vi "Exponential Smooth.vi"(10 "Smoothing Factor":dbl=0.1, 11 "Input Value":dbl) -> (3 "Smoothed Value":dbl)   [LabVIEW 2011]
doc: "Exponential smoothing weights the input value against the previous smoothing value.\n\nTODO: possible improvement: when there has been a long string of NaN inputs, we should probably disregard the old smoothed value and begin afresh."
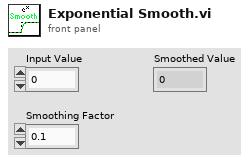
[diagram p1: front panel]
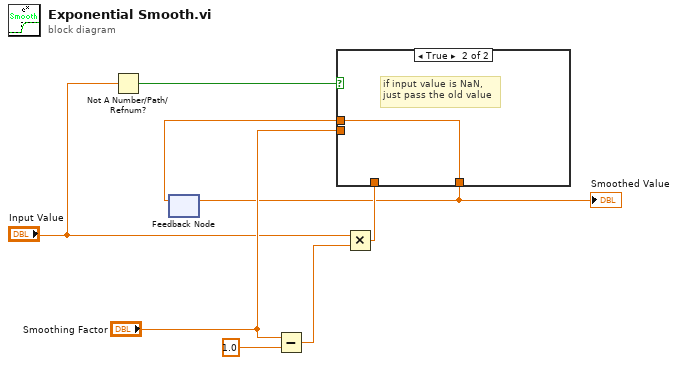
[diagram p0: block diagram]
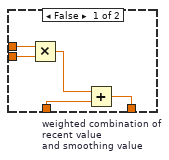
[diagram p2: hidden frame]
diagram:
  n1 = Not A Number/Path/Refnum?(number/path/refnum="Input Value") -> (NaN/Path/Refnum?=w1:bool)
  n2 = feedback #1() -> (w3:dbl)  [unwired: 1 in]
  n3 = Subtract(x="Smoothing Factor", y=1.0) -> (x-y=w8:dbl)
  n4 = Multiply(x="Input Value", y=w8) -> (x*y=w6:dbl)
  n5 = case shown="True" w1 {
    tunnel: "Smoothing Factor" -> [w13 _]
    tunnel: w6 -> [w12 _]
    tunnel: [w11 w14] -> w5
    tunnel: w3 -> [w10 w14]
    frame False {
      n6 = Multiply(x=w10, y=w13) -> (x*y=w9:dbl)
      n7 = Add "weighted combination of\nrecent value\nand smoothing value"(x=w9, y=w12) -> (x+y=w11:dbl)
    }
    frame True {
      # "if input value is NaN, \njust pass the old value"
    }
  }
  "Smoothed Value" <- w5
  n8 = feedback-in #1(w5) -> ()
